vi "Read Count Measurement (Serial Bus - UART).vi"(8 "error in (no error)":errorcluster, 10 "Serial Bus Name (1: Serial Bus 1)":i32(ring)=1 items=["Serial Bus 1"=1, "Serial Bus 2"=2], 11 "VISA resource name":refnum<visa-resource-name>) -> (0 "error out":errorcluster, 1 "Tx Frame Count":dbl, 2 "Rx Frame Count":dbl, 3 "VISA resource name out":refnum<visa-resource-name>, 5 "Error Frame Count":dbl)   [LabVIEW 2016, in "Agilent 2000 3000 X-Series.lvlib"]
doc: "Returns the measurement of serial bus - UART."
uses:
  Agilent 2000 3000 X-Series.lvlib
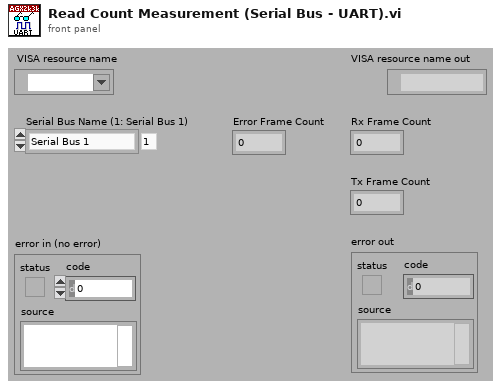
[diagram p1: front panel]
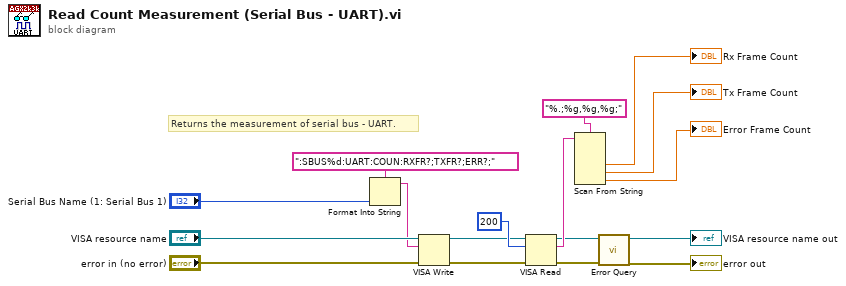
[diagram p0: block diagram]
diagram:
  # "Returns the measurement of serial bus - UART."
  n1 = Format Into String(format string=":SBUS%d:UART:COUN:RXFR?;TXFR?;ERR?;", "Serial Bus Name (1: Serial Bus 1)") -> (resulting string=w9:string)  [unwired: 2 in, 1 out]
  n2 = VISA Write(VISA resource name="VISA resource name", write buffer=w9, error in (no error)="error in (no error)") -> (VISA resource name out=w1:refnum<visa-resource-name>, error out=w4:errorcluster)  [unwired: 1 out]
  n3 = VISA Read(VISA resource name=w1, byte count=u32 200, error in (no error)=w4) -> (VISA resource name out=w2:refnum<visa-resource-name>, read buffer=w10:string, error out=w3:errorcluster)  [unwired: 1 out]
  n4 = Scan From String(format string="%.;%g,%g,%g;", input string=w10) -> (output 1=→"Rx Frame Count":dbl, output 2=→"Tx Frame Count":dbl, output 3=→"Error Frame Count":dbl)  [unwired: 2 in, 6 out]
  n5 = call "Error Query.vi"("error in (no error)"=w3, "VISA resource name"=w2) -> ("error out"=→"error out":errorcluster, "VISA resource name out"=→"VISA resource name out":refnum<visa-resource-name>)  [unwired: 8 out]
